vi "SetValue.vi"(0 "VI Reference":refnum<vi>, 5 "Control Name":string, 7 "Control Value":variant, 11 "error in":errorcluster) -> (4 "VI Reference out":refnum<vi>, 15 "error out":errorcluster)   [LabVIEW 2016]
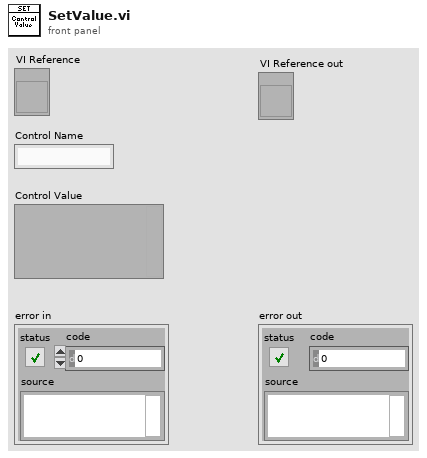
[diagram p1: front panel]
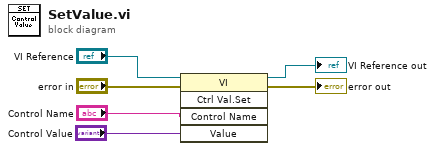
[diagram p0: block diagram]
diagram:
  n1 = invoke class="VI" method="Ctrl Val.Set"(reference="VI Reference", error in="error in", "Control Name"="Control Name", "Value"="Control Value") -> (reference out=→"VI Reference out":refnum<vi>, error out=→"error out":errorcluster)  [unwired: 1 in, 3 out]
